vi "target - single rate.vi"() -> ()   [LabVIEW 2013]
uses:
  <vilib>/Platform/TimedLoop/XDataNode/timing_clust.ctl
  <vilib>/Platform/TimedLoop/XDataNode/nitl_modes.ctl
  <vilib>/Platform/TimedLoop/XDataNode/wakeup.ctl
  <vilib>/Rock Robotics/SystemInterfaces/DIO/FPGA_DIOChannel.ctl
  <vilib>/Rock Robotics/SystemInterfaces/AI/FPGA_AIGyroChannel.ctl
  <vilib>/Rock Robotics/SystemInterfaces/DIO/FPGA_DIOPWMChannel.ctl
  <vilib>/Rock Robotics/WPI/SafetyOutput/WPI_SafetyOutputConfigMenu.ctl
  <vilib>/Rock Robotics/WPI/Joystick/WPI_JoystickDeviceEnum.ctl
  Program Files (x86)/National Instruments/LabVIEW 2013/examples/FRC/I2C/ADXL345 I2C/Driver/ADXL345 I2C Range.ctl
  Program Files (x86)/National Instruments/LabVIEW 2013/examples/FRC/I2C/ADXL345 I2C/Driver/ADXL345 I2C Axis.ctl
  <vilib>/Rock Robotics/WPI/Counter/WPI_CounterDigitalInputToDigitalSource.vi
  <vilib>/Rock Robotics/WPI/MotorControl/WPI_MotorControlOpen Victor.vi
  <vilib>/Rock Robotics/WPI/MotorControl/WPI_MotorControlOpen Jaguar.vi
  <vilib>/Rock Robotics/WPI/RobotDrive/WPI_RobotDriveOpen4MotorWithExistingMotors.vi
  <vilib>/Rock Robotics/WPI/RobotDrive/WPI_RobotDriveArcadeDrive_Standard(NoSaturation).vi
  <vilib>/Platform/TimedLoop/XDataNode/XDataNode.xnode
  <vilib>/Platform/TimedLoop/XDataNode/XDNodeRunTimeDep.lvlib
panel:
  out "Direction":dbl(knob)
  out "Velocity":dbl
  in  "Servo":i32(knob) max=360 step=1
  out "Battery Voltage":dbl
  in  "Joystick enbled":bool
  out "Acceleration":dbl
  out "Pantograph":i16[](graph)
  in  "Left axis":dbl(slide) step=0.1 scale=-1.0..1.0
  in  "Right axis":dbl(slide) step=0.1 scale=-1.0..1.0
  in  "Wheel diameter":dbl=1.0
  out "Current angle":dbl
  out "Distance":dbl
  out "Revolutions":dbl
  in  "Reset Gyro":bool
  in  "Reset Encoder":bool
  out "Encoder Rate":dbl
  out "Gyro":dbl(knob)
  in  "stop":bool
  # "Drive Motors"
  # "Encoder"
  # "Motion"
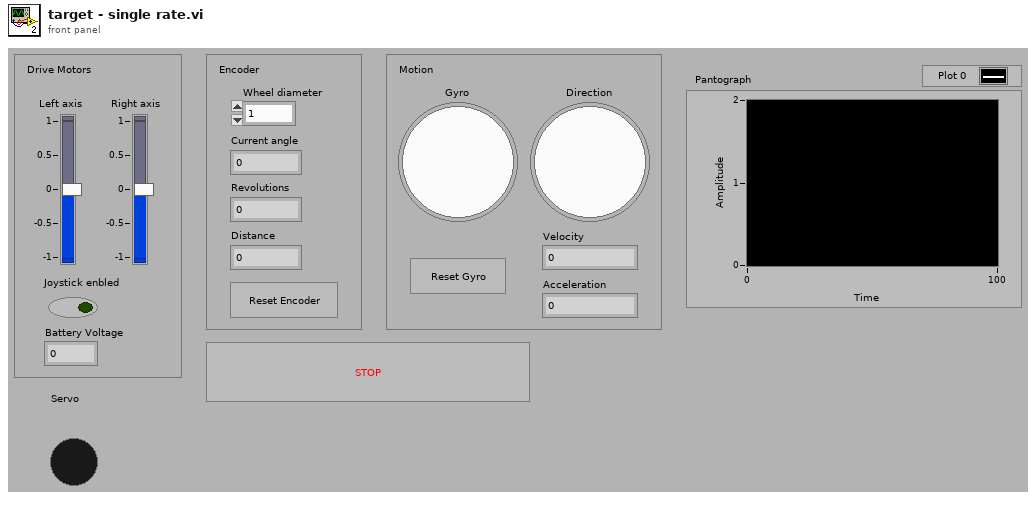
[diagram p1: front panel]
types:
  T1 = typedef "FPGA_DIOPWMChannel.ctl" = enum8{"PWM 1", "PWM 2", "PWM 3", "PWM 4", "PWM 5", "PWM 6", "PWM 7", "PWM 8", "PWM 9", "PWM 10", "Invalid"}
  T2 = typedef "ADXL345 I2C Range.ctl" = u8
  T3 = typedef "WPI_JoystickDeviceEnum.ctl" = enum16{"USB 1", "USB 2", "USB 3", "USB 4", "Kinect 1", "Kinect 2"}
  T4 = typedef "WPI_SafetyOutputConfigMenu.ctl" = enum16{"Enable", "Disable"}
  T5 = typedef "FPGA_AIGyroChannel.ctl" = enum8{"AI 1", "AI 2", "Invalid"}
  T6 = typedef "FPGA_DIOChannel.ctl" = enum8{"DIO 1", "DIO 2", "DIO 3", "DIO 4", "DIO 5", "DIO 6", "DIO 7", "DIO 8", "DIO 9", "DIO 10", "DIO 11", "DIO 12", "DIO 13", "DIO 14", "Invalid"}
  T7 = typedef "WPI_MotorControlDeviceRef.ctl" = cluster{"DeviceStatus":errorcluster, "Type":enum16{"PWM", "CAN"}, "PWM":cluster{"Digital Module":T8, "PWM Channel":T1, "DeadBand":T9}, "CAN":cluster{"Device Number":u8, "Control Mode":T10, "Semaphore":T11, "Max Vout":dbl}, "Invert":bool, "TransformRef":T12, "InvTransformRef":T12}
  T8 = typedef "FPGA_TypedefDigitalModule.ctl" = enum16{"Digital Module 1", "Digital Module 2"}
  T9 = typedef "WPI_PWMDeadband.ctl" = cluster{"Name":string, "maxPositivePwm":i32, "minPositivePwm":i32, "centerPwm":i32, "maxNegativePwm":i32, "minNegativePwm":i32, "angularRange":u16}
  T10 = typedef "WPI_CANJaguar_ControlMode.ctl" = enum8{"Percent VBus", "Current", "Speed", "Position", "Voltage"}
  T11 = typedef "Semaphore RefNum" = refnum<k1>
  T12 = typedef "WPI_PWMTransform_ConPane.ctl" = refnum<vi>
  T13 = typedef "WPI_DigitalInputDevRef.ctl" = cluster{"DevStatus":errorcluster, "DIO Channel":T6, "Digital Module":T8}
  T14 = typedef "WPI_GyroDevRef.ctl" = cluster{"DevStatus":errorcluster, "Analog Module":T15, "Analog Channel":T16, "Offset":dbl, "Gain (VoltsPerDegree/Second)":dbl}
  T15 = typedef "FPGA_TypedefAnalogModule.ctl" = enum16{"Analog Module 1", "Analog Module 2"}
  T16 = typedef "FPGA_AIChannel.ctl" = enum8{"AI 1", "AI 2", "AI 3", "AI 4", "AI 5", "AI 6", "AI 7", "AI 8", "Invalid"}
  T17 = typedef "FPGA_CounterEncoderSourceConvertionLVSourceType.ctl" = cluster{"DevStatus":errorcluster, "AnalogTriggerMode?":bool, "DigitalMode":cluster{"Digital Module":T8, "DIO Channel":T18}, "AnalogTriggerMode":cluster{"AnalogTriggerIndex":T19, "OutputType":T20}}
  T18 = typedef "FPGA_DIODigitalSourceChannel.ctl" = enum8{"DIO 1", "DIO 2", "DIO 3", "DIO 4", "DIO 5", "DIO 6", "DIO 7", "DIO 8", "DIO 9", "DIO 10", "DIO 11", "DIO 12", "DIO 13", "DIO 14", "Disabled"}
  T19 = typedef "FPGA_AnalogTriggerIndex.ctl" = enum8{"Trig 0", "Trig 1", "Trig 2", "Trig 3", "Trig 4", "Trig 5", "Trig 6", "Trig 7", "Invalid"}
  T20 = typedef "FPGA_AnalogTriggerOutType.ctl" = enum16{"InWindow", "TriggerState", "Rising", "Falling"}
  T21 = typedef "WPI_EncoderDevRef.ctl" = cluster{"DevStatus":errorcluster, "EncoderIndex":T22, "CounterIndex":T23, "DistancePerCount":dbl, "Decoding Type":T24}
  T22 = typedef "FPGA_EncoderIdx.ctl" = enum8{"Enc 0", "Enc 1", "Enc 2", "Enc 3", "Invalid"}
  T23 = typedef "FPGA_CounterCtrSystemIndex.ctl" = enum8{"Ctr 0", "Ctr 1", "Ctr 2", "Ctr 3", "Ctr 4", "Ctr 5", "Ctr 6", "Ctr 7", "Invalid"}
  T24 = typedef "WPI_EncoderType.ctl" = enum16{"1x", "2x", "4x"}
  T25 = typedef "WPI_RobotDriveDevRef.ctl" = cluster{"DevStatus":errorcluster, "Motors[]":T7[], "Square Inputs":bool, "Max Output":dbl, "Isochronous":bool}
  T26 = typedef "XDNodeRunTimeDep.lvlib/timing_clust.ctl" = cluster{"Expected End [f-1]":u64, "Actual End [f-1]":u64, "Finished Late? [f-1]":bool, "Expected End [i-1]":u64, "Actual End [i-1]":u64, "Finished Late? [i-1]":bool, "Expected Start [i]":u64, "Actual Start [i]":u64, "Expected Start [f]":u64, "Actual Start [f]":u64, "Source Name":string, "Structure Name":string, "Period":i64, "Deadline":i64, "Offset":i64, "Start":i64, "Priority":i32, "Timeout":i32, "Mode":T27, "Wakeup Reason":T28, "Error":errorcluster, "Source Type":string, "Secondary Source Type":string, "Global End Time":u64, "Global Start Time":u64, "Frame Duration":u64, "Iteration Duration":u64, "Assigned CPU":i32, "I/O Scan Engine Mode":u32}
  T27 = typedef "XDNodeRunTimeDep.lvlib/nitl_modes.ctl" = enum32{"No Change", "Process missed periods, maintain original phase", "Discard missed periods, maintain original phase", "Process missed periods, ignore original phase", "Discard missed periods, ignore original phase"}
  T28 = typedef "XDNodeRunTimeDep.lvlib/wakeup.ctl" = enum32{"Normal", "Aborted", "Asynchronous wakeup", "Timing source error", "Timed loop error", "Timeout"}
  T29 = typedef "WPI_I2CDevRef.ctl" = cluster{"DevStatus":errorcluster, "Digital Module":T8, "Device Address":u8}
  T30 = typedef "WPI_JoystickDevRef.ctl" = cluster{"Device":T3}
  T31 = typedef "WPI_ServoDeviceRef.ctl" = cluster{"DeviceStatus":errorcluster, "Digital Module":T8, "PWM Channel":T1, "DeadBand":T9}
  T32 = typedef "ADXL345 I2C Axis.ctl" = u8
  T33 = cluster{"axis 1 (x)":dbl, "axis 2 (y)":dbl, "axis 3 (throttle)":dbl, "axis 4":dbl, "axis 5":dbl, "axis 6":dbl}
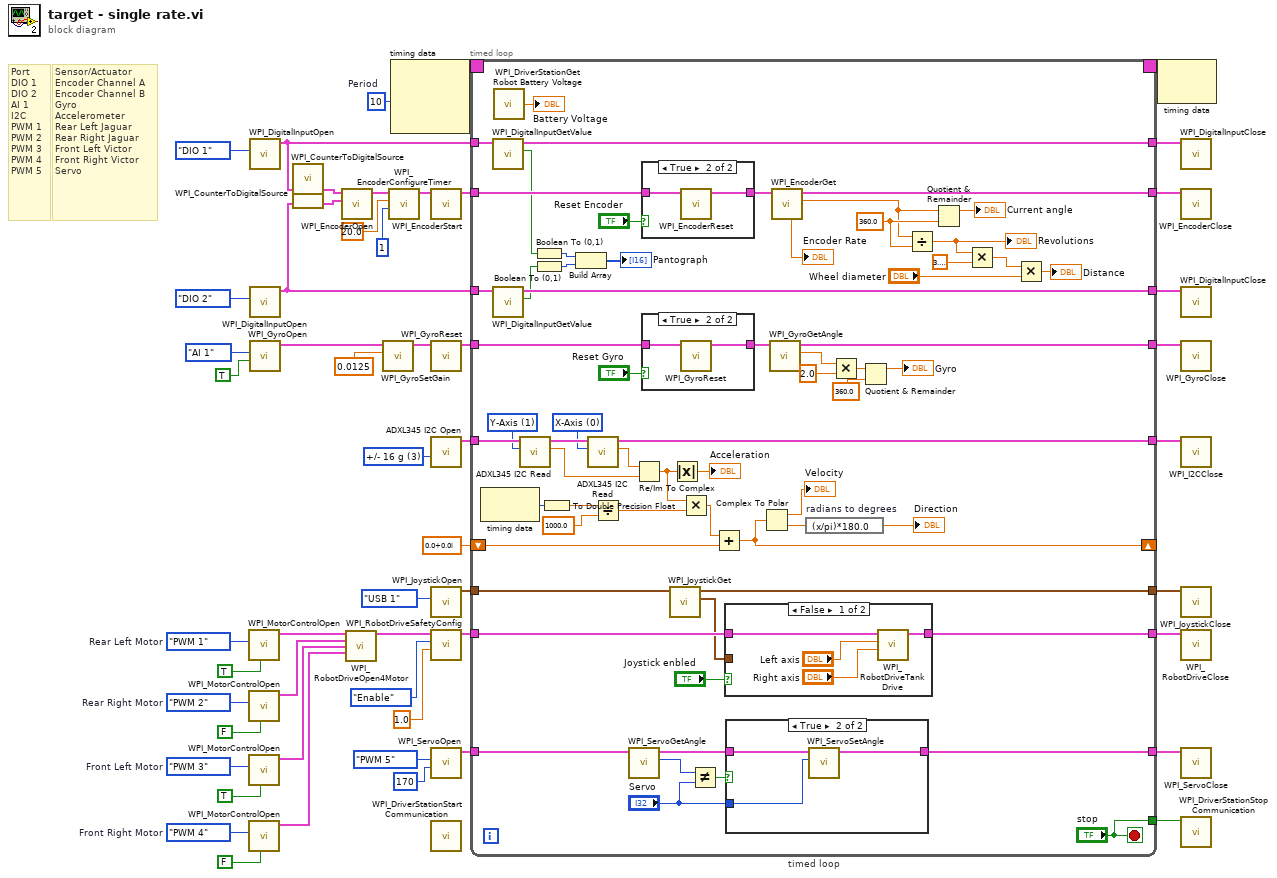
[diagram p0: block diagram]
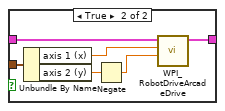
[diagram p3: hidden frame]
diagram:
  w12 = T2 3 items=["+/- 2 g", "+/- 4 g", "+/- 8 g", "+/- 16 g"] ("Range")
  w25 = FPGA_DIOPWMChannel."PWM 4"  # Front Right Motor
  w26 = FPGA_DIOPWMChannel."PWM 3"  # Front Left Motor
  w27 = FPGA_DIOPWMChannel."PWM 2"  # Rear Right Motor
  w24 = FPGA_DIOPWMChannel."PWM 1"  # Rear Left Motor
  w51 = i64 10  # Period
  # "Sensor/Actuator\nEncoder Channel A\nEncoder Channel B\nGyro\nAccelerometer\nRear Left Jaguar\nRear Right Jaguar\nFront Left Victor\nFront Right Victor\nServo"
  # "Port\nDIO 1\nDIO 2\nAI 1\nI2C\nPWM 1\nPWM 2\nPWM 3\nPWM 4\nPWM 5"
  n1 = call-poly <vilib>:"WPI_MotorControlOpen.vi"("Invert"=TRUE, "PWM Channel"=w24) -> ("MotorControlDeviceRef"=w20:T7)  [unwired: 8 in, 1 out]
  n2 = call-poly <vilib>:"WPI_MotorControlOpen.vi"("Invert"=FALSE, "PWM Channel"=w27) -> ("MotorControlDeviceRef"=w19:T7)  [unwired: 8 in, 1 out]
  n3 = call-poly <vilib>:"WPI_MotorControlOpen.vi"("Invert"=TRUE, "PWM Channel"=w26) -> ("MotorControlDeviceRef"=w18:T7)  [unwired: 8 in, 1 out]
  n4 = call-poly <vilib>:"WPI_MotorControlOpen.vi"("Invert"=FALSE, "PWM Channel"=w25) -> ("MotorControlDeviceRef"=w17:T7)  [unwired: 8 in, 1 out]
  n5 = call <vilib>:"WPI_DigitalInputOpen.vi"("DIO Channel"=FPGA_DIOChannel."DIO 1") -> ("DigitalInputDevRef"=w43:T13)  [unwired: 9 in, 1 out]
  n6 = call <vilib>:"WPI_DigitalInputOpen.vi"("DIO Channel"=FPGA_DIOChannel."DIO 2") -> ("DigitalInputDevRef"=w44:T13)  [unwired: 9 in, 1 out]
  n7 = call <vilib>:"WPI_GyroOpen.vi"("Calibrate On Open"=TRUE, "Analog Channel"=FPGA_AIGyroChannel."AI 1") -> ("GyroDevRef"=w36:T14)  [unwired: 7 in, 2 out]
  n8 = call-poly <vilib>:"WPI_CounterToDigitalSource.vi"("DigitalInputDevRef"=w43) -> ("Digital Source"=w46:T17)  [unwired: 6 in]
  n9 = call-poly <vilib>:"WPI_CounterToDigitalSource.vi"("DigitalInputDevRef"=w44) -> ("Digital Source"=w45:T17)  [unwired: 6 in]
  n10 = call <vilib>:"WPI_EncoderOpen.vi"("BSource"=w45, "ASource"=w46) -> ("EncoderDevRef"=w34:T21)  [unwired: 8 in, 1 out]
  n11 = call-poly <vilib>:"WPI_RobotDriveOpen4Motor.vi"("Rear Left Motor Dev Ref"=w20, "Rear Right Motor Dev Ref"=w19, "Front Left Motor Dev Ref"=w18, "Front Right Motor Dev Ref"=w17) -> ("RobotDriveDevRef"=w22:T25)  [unwired: 10 in, 1 out]
  n12 = call <vilib>:"WPI_GyroSetGain.vi"("Gain (VoltsPerDegree/Second)"=0.0125, "GyroDevRef"=w36) -> ("GyroDevRef"=w9:T14)  [unwired: 1 in, 8 out]
  n13 = call <vilib>:"WPI_EncoderConfigureTimer.vi"("Number Samples to Average"=u8 1, "Minimum Rate"=20.0, "EncoderDevRef"=w34) -> ("EncoderDevRef"=w33:T21)  [unwired: 1 in, 7 out]
  n14 = node-c288(w51) -> (w53:T26)  [unwired: 2 out]
  n15 = call <vilib>:"WPI_EncoderStart.vi"("EncoderDevRef"=w33) -> ("EncoderDevRef"=w39:T21)  [unwired: 9 in, 1 out]
  n16 = call <vilib>:"WPI_GyroReset.vi"("GyroDevRef"=w9) -> ("GyroDevRef"=w8:T14)  [unwired: 9 in, 1 out]
  n17 = call "ADXL345 I2C Open.vi"("Range"=w12) -> ("I2CDevRef"=w11:T29)  [unwired: 3 in, 7 out]
  n18 = call <vilib>:"WPI_JoystickOpen.vi"("JoystickDevice"=WPI_JoystickDeviceEnum."USB 1") -> ("JoystickDevRef"=w14:T30)  [unwired: 10 in]
  n19 = call <vilib>:"WPI_RobotDriveSafetyConfig.vi"("timeout (s)"=1.0, "mode"=WPI_SafetyOutputConfigMenu."Enable", "RobotDriveDevRef"=w22) -> ("RobotDriveDevRef"=w21:T25)  [unwired: 7 in, 1 out]
  n20 = call <vilib>:"WPI_ServoOpen.vi"("Angular Range"=u16 170, "PWM Channel"=FPGA_DIOPWMChannel."PWM 5") -> ("ServoDeviceRef"=w6:T31)  [unwired: 8 in, 1 out]
  n21 = call <vilib>:"WPI_DriverStationStart Communication.vi"() -> ()  [unwired: 1 in, 11 out]
  n22 = timed-loop "timed loop" {
    timing: w53 -> [_]
    timing-out: [_] -> w52
    tunnel: [w117] -> _
    tunnel: w43 -> [w117]
    tunnel: w44 -> [w116]
    tunnel: [w113] -> w40
    tunnel: [w95] -> w41
    tunnel: w8 -> [w105]
    tunnel: [w112] -> w47
    tunnel: w39 -> [w110]
    tunnel: [w97] -> w42
    tunnel: ["stop"] -> w38
    tunnel: w21 -> [w88]
    tunnel: [w68] -> w15
    tunnel: w14 -> [w89]
    tunnel: [w79] -> w10
    tunnel: w11 -> [w56]
    tunnel: w6 -> [w78]
    tunnel: [w74] -> w4
    tunnel: [w72] -> w3
    shift-right: [w60] -> _
    shift-left: cdb 0.0+0.0i ("x") -> [w61]
    stop <- "stop" stop-if-true
    w84 = T32 0 items=["X-Axis", "Y-Axis", "Z-Axis"] ("Axis")
    w55 = T32 1 items=["X-Axis", "Y-Axis", "Z-Axis"] ("Axis")
    w103 = 360.0 ("y")
    n23 = node-c288() -> (w58:i64)  [unwired: 1 out]
    n24 = call <vilib>:"WPI_DigitalInputGetValue.vi"("DigitalInputDevRef"=w117) -> ("Value"=w107:bool, "DigitalInputDevRef"=w95:T13)  [unwired: 8 in, 1 out]
    n25 = call <vilib>:"WPI_DigitalInputGetValue.vi"("DigitalInputDevRef"=w116) -> ("Value"=w94:bool, "DigitalInputDevRef"=w113:T13)  [unwired: 8 in, 1 out]
    n26 = call <vilib>:"WPI_DriverStationGet Robot Battery Voltage.vi"() -> ("robot battery voltage"=→"Battery Voltage":dbl)  [unwired: 14 in, 1 out]
    n27 = call "ADXL345 I2C Read.vi"("Axis"=w55, "I2CDevRef"=w56) -> ("Acceleration"=w65:dbl, "I2CDevRef Out"=w85:T29)  [unwired: 1 in, 7 out]
    n28 = Boolean To (0,1)(Boolean=w107) -> (0, 1=w115:i16)
    n29 = Boolean To (0,1)(Boolean=w94) -> (0, 1=w114:i16)
    n30 = To Double Precision Float(number=w58) -> (double precision float=w71:dbl)
    n31 = Build Array(w115, w114) -> (→"Pantograph":i16[])
    n32 = call "ADXL345 I2C Read.vi"("Axis"=w84, "I2CDevRef"=w85) -> ("Acceleration"=w66:dbl, "I2CDevRef Out"=w79:T29)  [unwired: 1 in, 7 out]
    n33 = Divide(x=w71, y=1000.0) -> (x/y=w69:dbl)
    n34 = call <vilib>:"WPI_ServoGetAngle.vi"("ServoDeviceRef"=w78) -> ("ServoDeviceRef"=w75:T31, "Angle"=w77:u16)  [unwired: 7 in, 1 out]
    n35 = Re/Im To Complex(1:w65, 2:w66) -> (0:w54:cdb)
    n36 = case shown="True" "Reset Encoder" {
      tunnel: w110 -> [w137 w139]
      tunnel: [w137 w138] -> w109
      frame False {
      }
      frame True {
        n37 = call <vilib>:"WPI_EncoderReset.vi"("EncoderDevRef"=w139) -> ("EncoderDevRef"=w138:T21)  [unwired: 1 in, 9 out]
      }
    }
    n38 = case shown="True" "Reset Gyro" {
      tunnel: w105 -> [w134 w136]
      tunnel: [w134 w135] -> w104
      frame False {
      }
      frame True {
        n39 = call <vilib>:"WPI_GyroReset.vi"("GyroDevRef"=w136) -> ("GyroDevRef"=w135:T14)  [unwired: 9 in, 1 out]
      }
    }
    n40 = call <vilib>:"WPI_JoystickGet.vi"("JoystickDevRef"=w89) -> ("Axes"=w87:T33, "JoystickDevRef"=w72:T30)  [unwired: 4 in, 1 out]
    n41 = Absolute Value(x=w54) -> (abs(x)=→"Acceleration":dbl)
    n42 = Multiply(x=w54, y=w69) -> (x*y=w62:cdb)
    n43 = Not Equal?(x=w77, y="Servo") -> (x != y?=w76:bool)
    n44 = Add(x=w62, y=w61) -> (x+y=w60:cdb)
    n45 = case shown="False" "Joystick enbled" {
      tunnel: w88 -> [w126 w129]
      tunnel: [w127 w128] -> w68
      tunnel: w87 -> [_ w133]
      frame False {
        n46 = call <vilib>:"WPI_RobotDriveTankDrive.vi"("Right axis value"="Right axis", "Left axis value"="Left axis", "RobotDriveDevRef"=w126) -> ("RobotDriveDevRef"=w127:T25)  [unwired: 6 in, 2 out]
      }
      frame True {
        n47 = Unbundle By Name(w133) -> ("axis 1 (x)"=w132:dbl, "axis 2 (y)"=w131:dbl)
        n48 = Negate(x=w131) -> (-x=w130:dbl)
        n49 = call-poly <vilib>:"WPI_RobotDriveArcadeDrive.vi"("Y axis value"=w130, "X axis value"=w132, "RobotDriveDevRef"=w129) -> ("RobotDriveDevRef"=w128:T25)  [unwired: 6 in, 2 out]
      }
    }
    n50 = case shown="True" w76 {
      tunnel: w75 -> [w120 w123]
      tunnel: [w120 w122] -> w74
      tunnel: "Servo" -> [_ w121]
      frame False {
      }
      frame True {
        n51 = call <vilib>:"WPI_ServoSetAngle.vi"("Angle"=w121, "ServoDeviceRef"=w123) -> ("ServoDeviceRef"=w122:T31)  [unwired: 8 in, 1 out]
      }
    }
    n52 = Complex To Polar(r * e^(i*theta)=w60) -> (r=→"Velocity":dbl, theta=w63:dbl)
    n53 = call <vilib>:"WPI_GyroGetAngle.vi"("GyroDevRef"=w104) -> ("Angle"=w91:dbl, "GyroDevRef"=w112:T14)  [unwired: 7 in, 2 out]
    n54 = call <vilib>:"WPI_EncoderGet.vi"("EncoderDevRef"=w109) -> ("Distance"=w96:dbl, "EncoderDevRef"=w97:T21, "Rate"=→"Encoder Rate":dbl)  [unwired: 5 in, 3 out]
    n55 = expression code="(x/pi)*180.0" "radians to degrees"(w63) -> (→"Direction":dbl)
    n56 = Multiply(x=w91, y=2.0) -> (x*y=w82:dbl)
    n57 = Quotient & Remainder(x=w82, y=360.0) -> (x-y*floor(x/y)=→"Gyro":dbl)  [unwired: 1 out]
    n58 = Divide(x=w96, y=w103) -> (x/y=w102:dbl)
    "Revolutions" <- w102
    n59 = Quotient & Remainder(x=w96, y=w103) -> (x-y*floor(x/y)=→"Current angle":dbl)  [unwired: 1 out]
    n60 = Multiply(x=w102, y=3.141592653589793) -> (x*y=w99:dbl)
    n61 = Multiply(x=w99, y="Wheel diameter") -> (x*y=→"Distance":dbl)
  }
  n62 = node-c288(w52) -> ()  [unwired: 1 out]
  n63 = call <vilib>:"WPI_DigitalInputClose.vi"("DigitalInputDevRef"=w41) -> ()  [unwired: 10 in, 1 out]
  n64 = call <vilib>:"WPI_EncoderClose.vi"("EncoderDevRef"=w42) -> ()  [unwired: 10 in, 1 out]
  n65 = call <vilib>:"WPI_DigitalInputClose.vi"("DigitalInputDevRef"=w40) -> ()  [unwired: 10 in, 1 out]
  n66 = call <vilib>:"WPI_GyroClose.vi"("GyroDevRef"=w47) -> ()  [unwired: 10 in, 1 out]
  n67 = call <vilib>:"WPI_I2CClose.vi"("I2CDevRef"=w10) -> ()  [unwired: 10 in, 1 out]
  n68 = call <vilib>:"WPI_JoystickClose.vi"("JoystickDevRef"=w3) -> ()  [unwired: 11 in]
  n69 = call <vilib>:"WPI_RobotDriveClose.vi"("RobotDriveDevRef"=w15) -> ()  [unwired: 10 in, 1 out]
  n70 = call <vilib>:"WPI_ServoClose.vi"("MotorControlDevRef"=w4) -> ()  [unwired: 10 in, 1 out]
  n71 = call <vilib>:"WPI_DriverStationStop Communication.vi"("StopCommunication"=w38) -> ()  [unwired: 1 in, 10 out]
